vi "test.IndexStringToEnum.vi"() -> ()   [LabVIEW 2017]
panel:
  out "Enum":variant=variant(enum16{"Input - 输入", "Output - 输出", "Record - 记录"} enum."Input - 输入")
  in  "String 2":string="2"
  out "Direction":T1(ring)
  in  "String":string="-2"
  out "data":T2(ring)=enum."-2 ___ 虚拟开关输入通道"
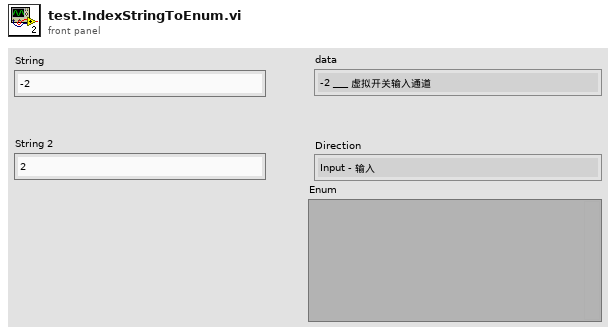
[diagram p1: front panel]
types:
  T1 = enum16{"Input - 输入", "Output - 输出", "Record - 记录"}
  T2 = enum16{"-4 ___ 虚拟开关输出通道", "-3 ___ 虚拟模拟输出通道", "-2 ___ 虚拟开关输入通道", "-1 ___ 虚拟模拟输入通道", "0 ___ 系统没有使用通道", "1 ___ 真实模拟输出通道", "2 ___ 真实开关输出通道", "3 ___ 真实模拟输入通道", "4 ___ 真实开关输入通道"}
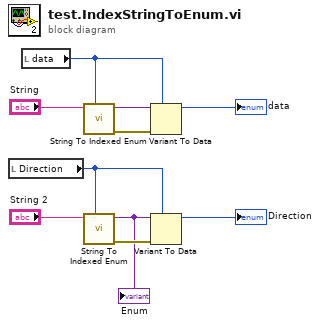
[diagram p0: block diagram]
diagram:
  n1 = local read "Direction"() -> (w5:T1)
  n2 = local read "data"() -> (w6:T2)
  n3 = call "String To Indexed Enum.vi"("Variant"=w6, "String"="String") -> ("error out"=w8:errorcluster, "Enum"=w9:variant)  [unwired: 8 in]
  n4 = call "String To Indexed Enum.vi"("Variant"=w5, "String"="String 2") -> ("error out"=w3:errorcluster, "Enum"=w2:variant)  [unwired: 8 in]
  "Enum" <- w2
  n5 = Variant To Data(error in=w8, type=w6, Variant=w9) -> (data=→"data":T2)  [unwired: 1 out]
  n6 = Variant To Data(error in=w3, type=w5, Variant=w2) -> (data=→"Direction":T1)  [unwired: 1 out]
